vi "PromptConfig.vi"(2 "error in (no error)":errorcluster, 3 "EpiWrapper in":refnum<class "EpiWrapper.lvclass">) -> (0 "error out":errorcluster, 1 "EpiWrapper out":refnum<class "EpiWrapper.lvclass">)   [LabVIEW 2012, in "EpiWrapper.lvclass"]
uses:
  EpiWrapper.lvclass
  EpiWrapper.lvclass/EpiWrapper.ctl
  Instruments.lvclass
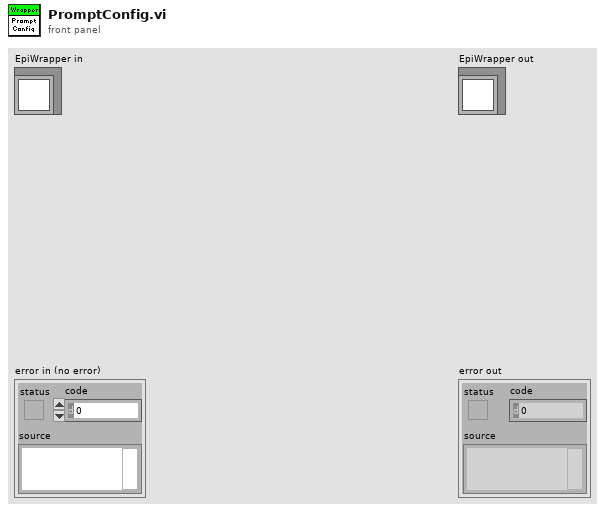
[diagram p1: front panel]
types:
  T1 = typedef "Config.ctl" = cluster{"IntTime":i32, "Samples":i32, "PowerMin":dbl, "KneeMin":dbl, "KneeMax":dbl, "BackgroundWl":dbl}
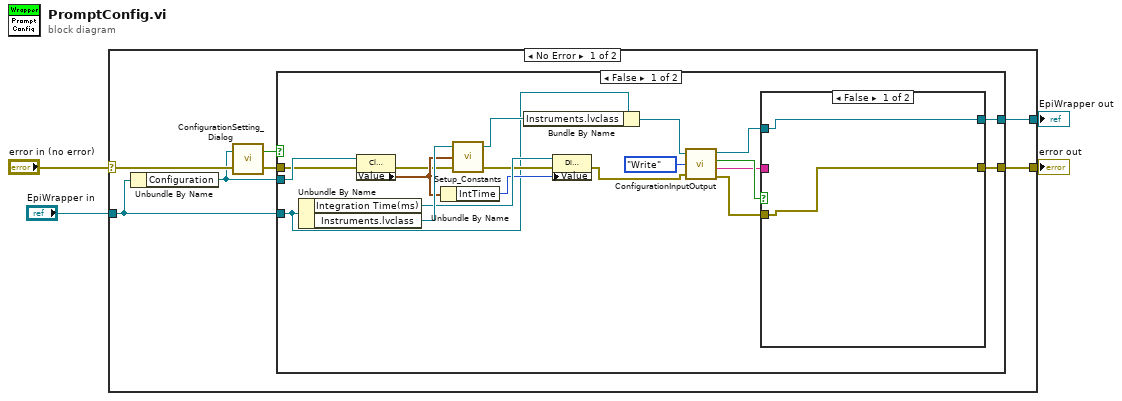
[diagram p0: block diagram]
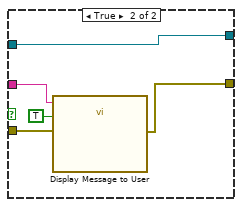
[diagram p2: hidden frame]
diagram:
  n1 = case shown="No Error" "error in (no error)" {
    selector: "error in (no error)" -> [w11 w41]
    tunnel: [w9 w41] -> w3
    tunnel: [w6 w40] -> w1
    tunnel: "EpiWrapper in" -> [w7 w40]
    frame No Error {
      n2 = Unbundle By Name(w7) -> ("Configuration"=w5:refnum<vi>)
      n3 = call "ConfigurationSetting_Dialog.vi"("error in (no error)"=w11, "Configuration"=w5) -> ("error out"=w8:errorcluster, "Cancelled?"=w10:bool)
      n4 = case shown="False" w10 {
        tunnel: [w15 w39] -> w9
        tunnel: w8 -> [w21 w39]
        tunnel: w7 -> [w25 w38]
        tunnel: [w13 w38] -> w6
        tunnel: w5 -> [w24 _]
        frame False {
          n5 = Unbundle By Name(w25) -> ("Integration Time(ms)"=w28:refnum<vi>, "Instruments.lvclass"=w30:refnum<class "Instruments.lvclass">)
          n6 = property class="Clust (strict)"(reference=w24, error in=w21) -> (error out=w22:errorcluster, "Value"=w23:T1)  [unwired: 1 out]
          n7 = Unbundle By Name(w23) -> ("IntTime"=w27:i32)
          n8 = call-dynamic "Setup_Constants.vi"("error in (no error)"=w22, "Config In"=w23, "Instruments in"=w30) -> ("error out"=w26:errorcluster, "Instruments out"=w29:refnum<class "Instruments.lvclass">)  [unwired: 1 in]
          n9 = Bundle By Name(cluster=w25, "Instruments.lvclass"=w29) -> (w20:refnum<class "EpiWrapper.lvclass">)
          n10 = property class="DigNum (strict)"(reference=w28, error in=w26, "Value"=w27) -> (error out=w18:errorcluster)  [unwired: 1 out]
          n11 = call-dynamic "ConfigurationInputOutput.vi"("EpiWrapper in"=w20, "Action"=enum16{"Read", "Write"}."Write", "error in (no error)"=w18) -> ("EpiWrapper out"=w14:refnum<class "EpiWrapper.lvclass">, "error?"=w17:bool, "message"=w12:string, "error out"=w16:errorcluster)
          n12 = case shown="False" w17 {
            tunnel: w16 -> [w31 w36]
            tunnel: [w31 w35] -> w15
            tunnel: w14 -> [w32 w34]
            tunnel: [w32 w34] -> w13
            tunnel: w12 -> [_ w33]
            frame False {
            }
            frame True {
              n13 = call "Display Message to User"("error in (no error)"=w36, "Enable"=TRUE, "Message"=w33) -> ("error out"=w35:errorcluster)  [unwired: 7 in, 1 out]
            }
          }
        }
        frame True {
        }
      }
    }
    frame Error {
    }
  }
  "error out" <- w3
  "EpiWrapper out" <- w1
